vi "Write State.vi"(8 "error in (no error)":errorcluster, 10 "State":enum16{"Kick", "Exit", "GoToBall", "BallToGoal"}(ring), 11 "AttackTacticVSS in":refnum<class "AttackTacticVSS.lvclass">) -> (0 "error out":errorcluster, 3 "AttackTacticVSS out":refnum<class "AttackTacticVSS.lvclass">)   [LabVIEW 2023, in "AttackTacticVSS.lvclass"]
uses:
  AttackTacticVSS.lvclass
  AttackTacticVSS.lvclass/AttackTacticVSS.ctl
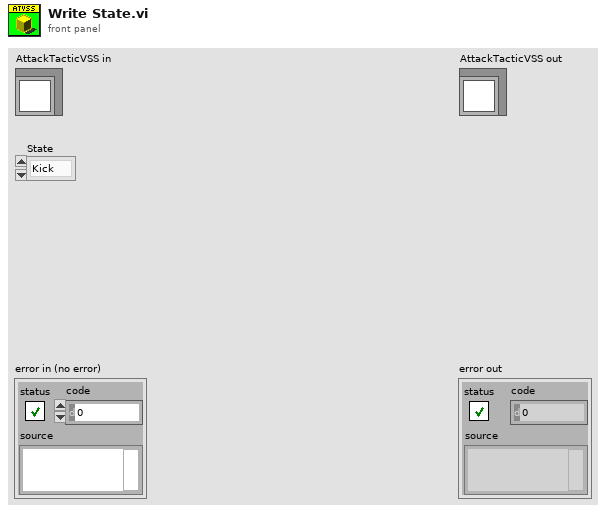
[diagram p1: front panel]
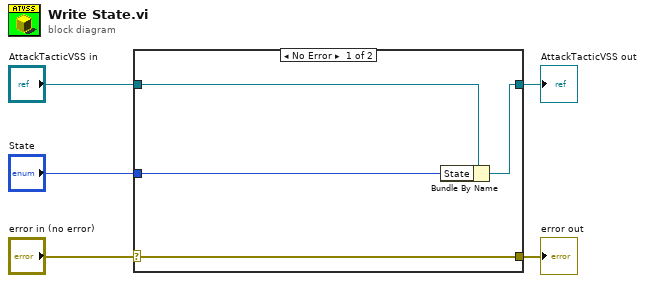
[diagram p0: block diagram]
diagram:
  n1 = case shown="No Error" "error in (no error)" {
    selector: "error in (no error)" -> [w9 w10]
    tunnel: [w9 w10] -> w4
    tunnel: [w7 w11] -> w2
    tunnel: "AttackTacticVSS in" -> [w8 w11]
    tunnel: "State" -> [w6 _]
    frame No Error {
      n2 = Bundle By Name(cluster=w8, "State"=w6) -> (w7:refnum<class "AttackTacticVSS.lvclass">)
    }
    frame Error {
    }
  }
  "error out" <- w4
  "AttackTacticVSS out" <- w2
